vi "ArmTuningPathGenerator.vi"() -> ()   [LabVIEW 2017]
panel:
  in  "Extension Motion Profile":dbl
  in  "Rotation Motion Profile":dbl
  in  "Reverse Button":bool
  in  "Go Button":bool
  in  "End Extension":dbl
  in  "Start Extension":dbl
  in  "End Angle":dbl
  in  "Start Angle":dbl
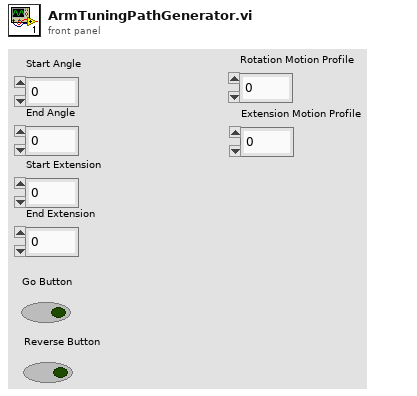
[diagram p1: front panel]
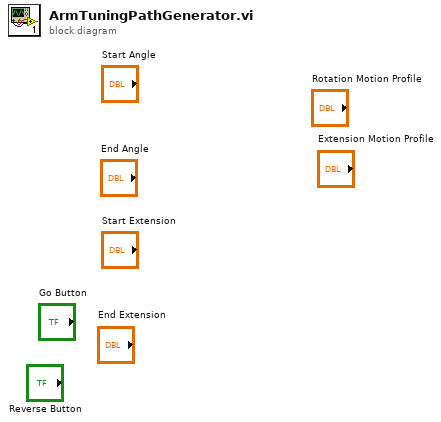
[diagram p0: block diagram]
diagram:
